vi "UART_Histograma.vi"() -> ()   [LabVIEW 2020]
uses:
  <vilib>/Instr/_visa.llb/VISA Configure Serial Port (Instr).vi
  <vilib>/ptbypt/NI_PtbyPt.lvlib
panel:
  in  "sample length":i32=10000
  out "Histogram Graph":T1(graph)
  in  "VISA resource name":refnum<visa-resource-name>
  out "String 2":string
  in  "stop":bool
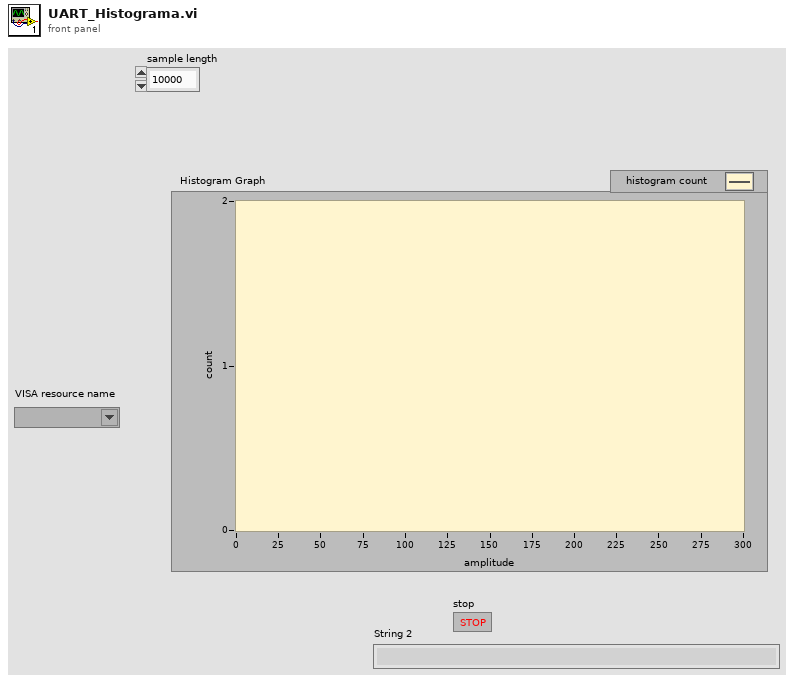
[diagram p1: front panel]
types:
  T1 = cluster{"X Values":dbl[], "Histogram: h(x)":i32[]}
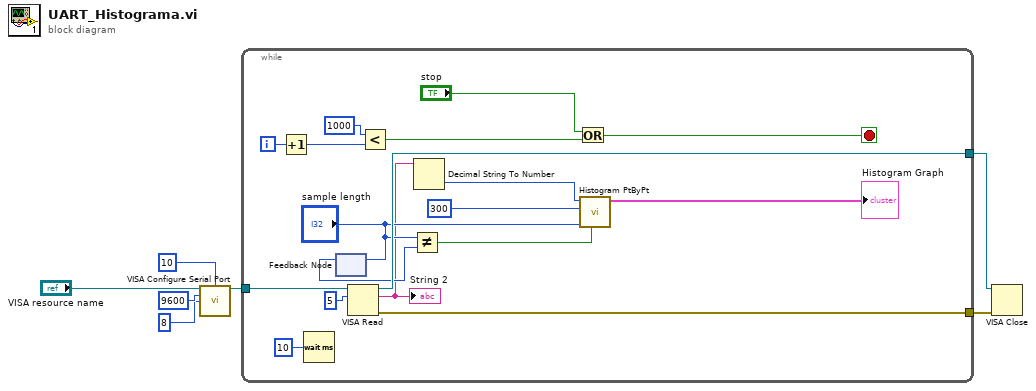
[diagram p0: block diagram]
diagram:
  n1 = call-poly "VISA Configure Serial Port"("VISA resource name"="VISA resource name", "termination char\n(0xA = '\\n' = LF)"=u8 10 ("termination char\n(0xA = '\\n' = LF)"), "baud rate (9600)"=u32 9600, "data bits (8)"=u16 8) -> ("VISA resource name out"=w4:refnum<visa-resource-name>)  [unwired: 10 in, 1 out]
  n2 = while {
    tunnel: w4 -> [w25]
    tunnel: [w23] -> w3
    tunnel: [w21] -> w2
    i -> [w14]
    stop <- w17 stop-if-true
    n3 = Increment(x=w14) -> (x+1=w13:i32)
    n4 = Wait (ms)(milliseconds to wait=u32 10) -> ()  [unwired: 1 out]
    n5 = feedback-in #1("sample length") -> ()
    n6 = feedback #1() -> (w12:i32)  [unwired: 1 in]
    n7 = VISA Read(VISA resource name=w25, byte count=u32 5) -> (VISA resource name out=w23:refnum<visa-resource-name>, read buffer=w8:string, error out=w21:errorcluster)  [unwired: 1 in, 1 out]
    "String 2" <- w8
    n8 = Less?(x=1000, y=w13) -> (x < y?=w15:bool)
    n9 = Not Equal?(x="sample length", y=w12) -> (x != y?=w11:bool)
    n10 = Decimal String To Number(string=w8) -> (number=w9:i32)  [unwired: 2 in, 1 out]
    n11 = Or(x="stop", y=w15) -> (x .or. y?=w17:bool)
    n12 = call <vilib>:"Histogram PtByPt.vi"("initialize"=w11, "sample length"="sample length", "intervals"=300, "x"=w9) -> ("Histogram Graph"=→"Histogram Graph":T1)  [unwired: 4 in, 3 out]
  }
  n13 = VISA Close(VISA resource name=w3, error in (no error)=w2) -> ()  [unwired: 1 out]
